vi "Send Data To Tree.vi"(8 "error in (no error)":errorcluster, 10 "Datas":string[][](table), 11 "Steps_Tree in":refnum<class "UI_Tree.lvclass">) -> (0 "error out":errorcluster, 3 "Steps_Tree out":refnum<class "UI_Tree.lvclass">)   [LabVIEW 2021, in "UI_Tree.lvlib" / "UI_Tree.lvclass"]
uses:
  UI_Tree.lvclass
  <vilib>/National Instruments/Tree Map/Tree Map Data.ctl
  UI_Tree.lvclass/UI_Tree.ctl
  <vilib>/National Instruments/Tree Map/API/List Roots.vi
  <vilib>/National Instruments/Tree Map/Utility/Into Tree Control Items.vi
  <vilib>/National Instruments/Tree Map/Tree Map.lvlib
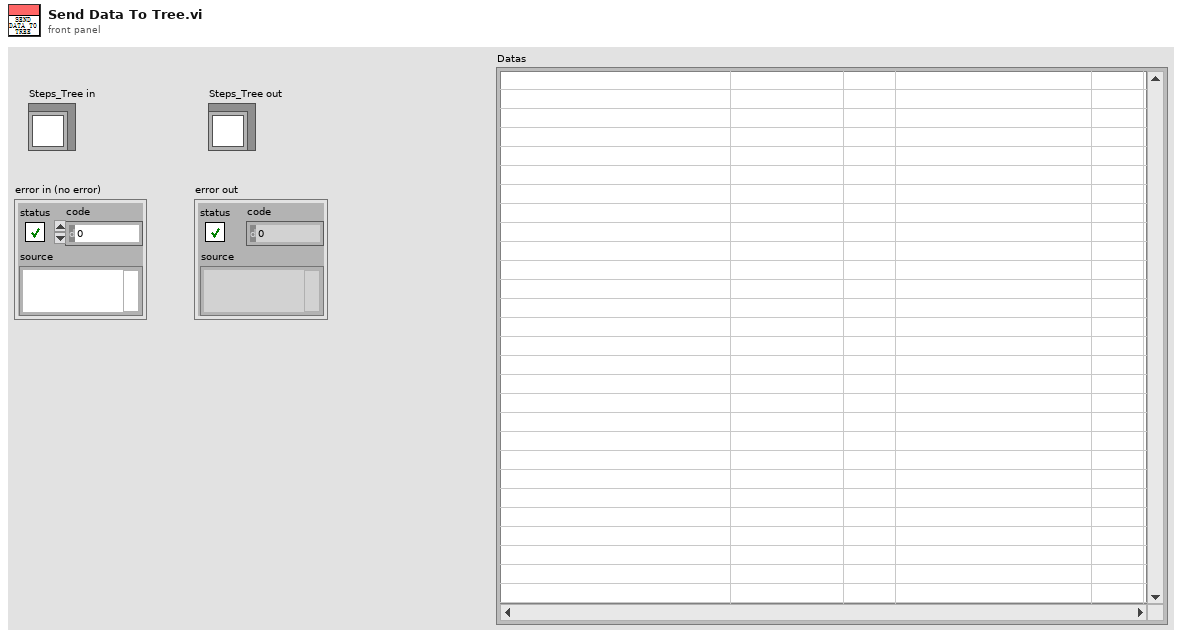
[diagram p1: front panel]
types:
  T1 = typedef "Tree Map.lvlib/Tree Map Data.ctl" = map{string, cluster{"Child Paths Set":set{string}, "Name":string, "Data":string, "Attributes":map{string, string}}}
  T2 = cluster{"Left Cell String":string, "Child Text":string[], "Child Tag":string, "Item Indent":i32, "Child Only?":bool, "Glyph Index":i32}[]
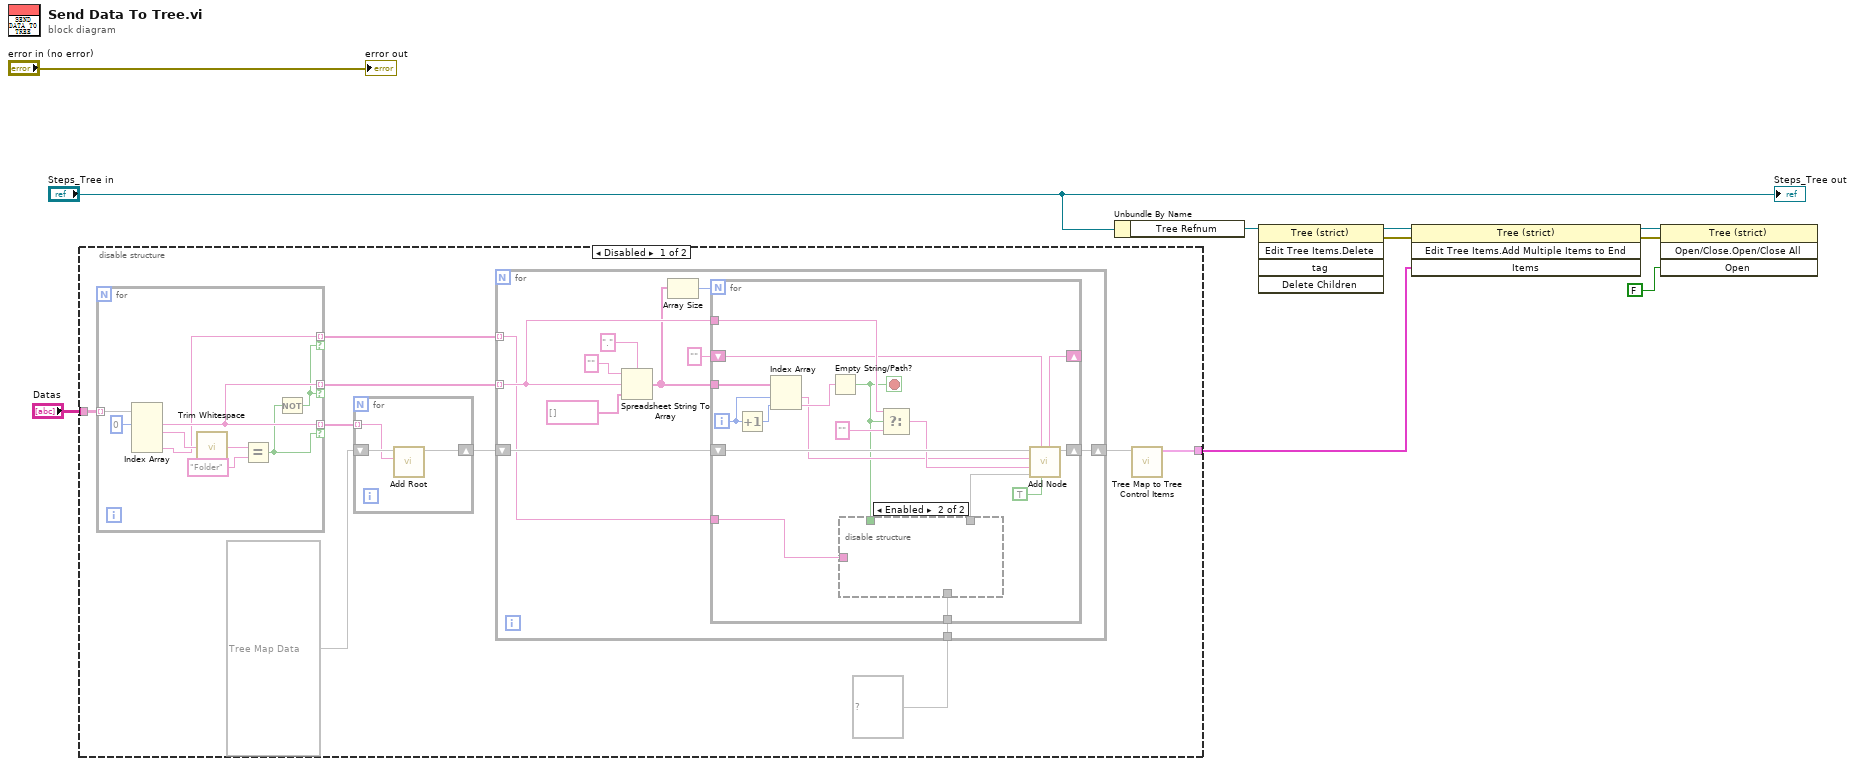
[diagram p0: block diagram]
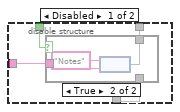
[diagram p2: hidden frame]
diagram:
  n1 = disable-structure shown="Disabled" {
    disable-tunnel: [w14 _] -> w7
    disable-tunnel: "Datas" -> [w11 _]
    frame Disabled {
      n2 = for {
        tunnel: w11 -> [w31] mode=indexing
        tunnel: [w26] -> w18 mode=indexing if=w25
        tunnel: [w26] -> w16 mode=indexing if=w23
        tunnel: [w24] -> w13 mode=indexing if=w23
        n3 = Index Array(array=w31, index #1=0 ("index")) -> (element #1=w26:string, element #2=w29:string, element #4=w24:string)  [unwired: 3 in, 1 out]
        n4 = call <vilib>:"Trim Whitespace.vi"("string"=w29) -> ("trimmed string"=w28:string)  [unwired: 1 in]
        n5 = Equal?(x=w28, y="Folder") -> (x = y?=w25:bool)
        n6 = Not(x=w25) -> (.not. x?=w23:bool)
      }
      n7 = for {
        shift-right: [w22] -> w17
        shift-left: T1 {} ("Tree Map Out") -> [w21]
        tunnel: w18 -> [w20] mode=indexing
        n8 = call <vilib>:"Add Root.vi"("New Root Name"=w20, "Tree Map In"=w21) -> ("Tree Map Out"=w22:T1)  [unwired: 8 in, 1 out]
      }
      n9 = for {
        shift-right: [w41] -> w15
        shift-left: w17 -> [w42]
        tunnel: w16 -> [w40] mode=indexing
        tunnel: w13 -> [w32] mode=indexing
        tunnel: map{string, string} {} ("Attributes") -> [w33]
        n10 = Spreadsheet String To Array(delimiter (Tab)=".", format string="", spreadsheet string=w40, array type (2D Dbl)=string[] [] ("Datas")) -> (array=w36:string[])
        n11 = Array Size(array=w36) -> (size(s)=w35:i32)
        n12 = for {
          N: w35 -> [_]
          shift-right: [w58] -> w41
          shift-left: w42 -> [w59]
          tunnel: w36 -> [w51]
          tunnel: w40 -> [w56]
          shift-right: [w53] -> _
          shift-left: "" ("New Node Path") -> [w52]
          tunnel: w33 -> [w45]
          tunnel: w32 -> [w43]
          i -> [w50]
          stop <- w46 stop-if-true
          n13 = Increment(x=w50) -> (x+1=w49:i32)
          n14 = Index Array(array=w51, index #1=w50, index #2=w49) -> (element #1=w47:string, element #2=w48:string)
          n15 = Empty String/Path?(string/path=w48) -> (empty?=w46:bool)
          n16 = disable-structure shown="Enabled" {
            disable-tunnel: w46 -> [w63 _]
            disable-tunnel: w45 -> [w62 _]
            disable-tunnel: [w61 _] -> w44
            disable-tunnel: w43 -> [w60 _]
            frame Disabled {
              n17 = case shown="True" w63 {
                tunnel: [w64 w67] -> w61
                tunnel: w62 -> [w64 _]
                tunnel: w60 -> [_ w66]
                frame False {
                }
                frame True {
                  n18 = node("Notes" ("key"), w66) -> (w67:map{string, string})
                }
              }
            }
            frame Enabled {
            }
          }
          n19 = Select(t=w56, s=w46, f="") -> (s? t:f=w55:string)
          n20 = call <vilib>:"Add Node.vi"("T: Ignore Repeat Root"=TRUE, "Parent Path"=w52, "Attributes"=w44, "Data"=w55, "New Node Name"=w47, "Tree Map In"=w59) -> ("Tree Map Out"=w58:T1, "New Node Path"=w53:string)  [unwired: 3 in, 1 out]
        }
      }
      n21 = call <vilib>:"Tree Map to Tree Control Items.vi"("Tree Map In"=w15) -> ("Tree Control Items"=w14:T2)  [unwired: 10 in]
    }
    frame Enabled {
    }
  }
  n22 = Unbundle By Name("Steps_Tree in") -> ("Tree Refnum"=w9:refnum<vi>)
  n23 = invoke class="Tree (strict)" method="Edit Tree Items.Delete"(reference=w9) -> (reference out=w8:refnum<vi>, error out=w5:errorcluster)  [unwired: 4 in, 3 out]
  n24 = invoke class="Tree (strict)" method="Edit Tree Items.Add Multiple Items to End"(reference=w8, error in=w5, "Items"=w7) -> (reference out=w3:refnum<vi>, error out=w4:errorcluster)  [unwired: 1 in, 2 out]
  n25 = invoke class="Tree (strict)" method="Open/Close.Open/Close All"(reference=w3, error in=w4, "Open"=FALSE ("Open?")) -> ()  [unwired: 1 in, 4 out]
  "error out" <- "error in (no error)"
  "Steps_Tree out" <- "Steps_Tree in"
